vi "浮点转CDAB整形cod.vi"(11 "浮点数":sgl[](array[numeric])) -> (3 "CDAB整形输出":u16[](array[numeric]) format="%04xH")   [LabVIEW 2016, in "斯坦道CODMn.lvlib"]
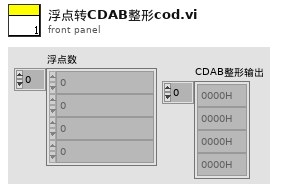
[diagram p1: front panel]
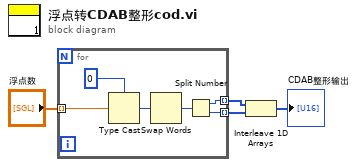
[diagram p0: block diagram]
diagram:
  n1 = for {
    tunnel: "浮点数" -> [w8] mode=indexing
    tunnel: [w7] -> w2 mode=indexing
    tunnel: [w6] -> w3 mode=indexing
    n2 = Type Cast(type=0, x=w8) -> (*(type *) &x=w5:i32)
    n3 = Swap Words(1:w5) -> (0:w10:i32)
    n4 = Split Number(x=w10) -> (hi(x)=w7:u16, lo(x)=w6:u16)
  }
  n5 = Interleave 1D Arrays(w2, w3) -> (→"CDAB整形输出":u16[])
